vi "3D curvature tensor algebra --V3.vi"(5 "error mode":T1, 6 "means":T2, 7 "2D tensor action":T4, 9 "3D curvature Matrix IN":T3, 11 "3D curvature tensor IN":T5={"curvature Matrix"=[[3.0, 1.0], [1.0, 4.0]], "eigenvs"=[4.618033988749895, 2.381966011250105], "Eigenvectors"=[[-0.8506508083520399+0.0i, -0.5257311121191335+0.0i], [0.5257311121191335+0.0i, -0.8506508083520399+0.0i]], "theta (rad)"=0.5535743588970453, "theta (deg)"=31.717474411461012, "Δs"=[4.618033988749895, 2.381966011250105], "δG/G"=0.5535743588970453, "Δlog(s)"=[4.618033988749895, 2.381966011250105], "inverse Matrix"=[[3.0, 1.0], [1.0, 4.0]], "noise T"=0.5535743588970453} {"noise T" format="%#_3f"; "inverse Matrix" format="%#_3p"; "Δlog(s)" scale=0.001..10.0; "δG/G" format="%#_3f"; "Δs" format="%#_2p"; "theta (deg)" format="%#_3p"; "curvature Matrix" format="%#_3p"; "eigenvs" format="%#_2f"; "Eigenvectors" format="%#_3p"; "theta (rad)" format="%#_3p"}) -> (1 "3D curvature Matrix OUT":T3, 3 "3D curvature tensor OUT":T5={"curvature Matrix"=[[3.0, 1.0], [1.0, 4.0]], "eigenvs"=[4.618033988749895, 2.381966011250105], "Eigenvectors"=[[-0.8506508083520399+0.0i, -0.5257311121191335+0.0i], [0.5257311121191335+0.0i, -0.8506508083520399+0.0i]], "theta (rad)"=0.5535743588970453, "theta (deg)"=31.717474411461012, "Δs"=[4.618033988749895, 2.381966011250105], "δG/G"=0.5535743588970453, "Δlog(s)"=[4.618033988749895, 2.381966011250105], "inverse Matrix"=[[3.0, 1.0], [1.0, 4.0]], "noise T"=0.5535743588970453} {"noise T" format="%#_3f"; "inverse Matrix" format="%#_3p"; "Δlog(s)" scale=0.001..10.0; "δG/G" format="%#_3f"; "Δs" format="%#_2p"; "theta (deg)" format="%#_3p"; "curvature Matrix" format="%#_3p"; "eigenvs" format="%#_2f"; "Eigenvectors" format="%#_3p"; "theta (rad)" format="%#_3p"})   [LabVIEW 2021]
uses:
  3D curvature tensor.ctl
  <vilib>/Analysis/Matrix/Datatypes/RealMatrix.ctl
  <vilib>/Analysis/Matrix/Datatypes/ComplexMatrix.ctl
  2D curvature tensor actions.ctl
  3-vec.ctl
  nanocal generate curvature ellipse -- action.ctl
  <vilib>/Analysis/7linalg.llb/Eigenvalue and Vectors Output Option.ctl
  <vilib>/Analysis/7linalg.llb/Real Eigenvalues and Vectors.vi
  <vilib>/Analysis/baseanly.llb/Real Inverse Matrix.vi
  <vilib>/Analysis/NI_AALBase.lvlib
  <vilib>/Analysis/NI_AALPro.lvlib
  <vilib>/Analysis/Matrix/NI_Matrix.lvlib
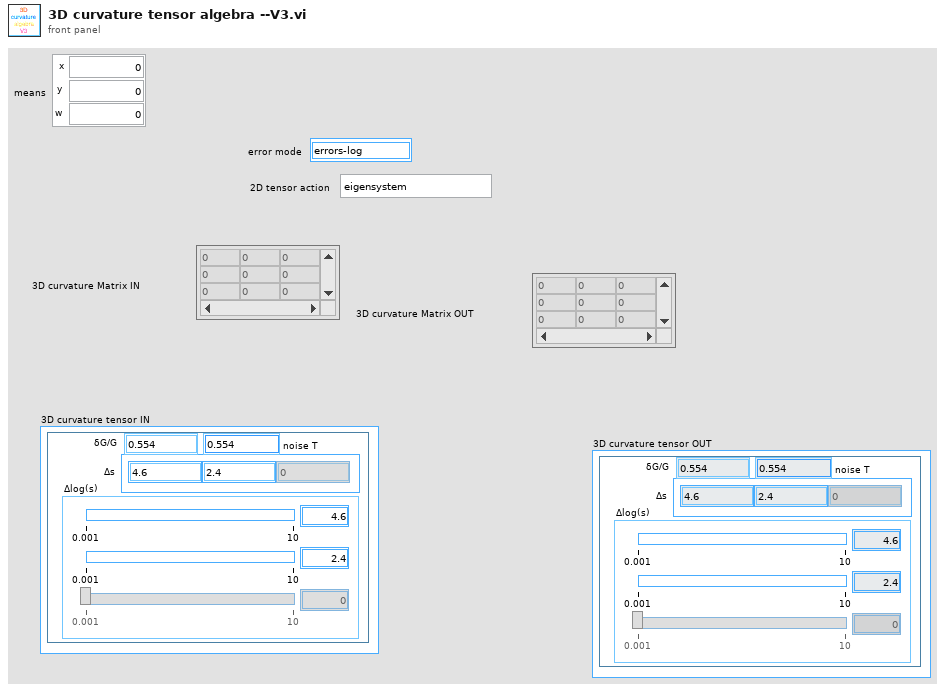
[diagram p1: front panel]
types:
  T1 = typedef "nanocal generate curvature ellipse -- action.ctl" = enum16{"errors-log", "errors-linear"}
  T2 = typedef "3-vec.ctl" = cluster{"x":dbl, "y":dbl, "w":dbl}
  T3 = typedef "NI_Matrix.lvlib/RealMatrix.ctl" = dbl[][]
  T4 = typedef "2D curvature tensor actions.ctl" = enum16{"eigensystem", "sigma", "set matrix", "inverse"}
  T5 = typedef "3D curvature tensor.ctl" = cluster{"curvature Matrix":T3, "eigenvs":dbl[], "Eigenvectors":T6, "theta (rad)":dbl, "theta (deg)":dbl, "Δs":dbl[], "δG/G":dbl, "Δlog(s)":dbl[], "inverse Matrix":T3, "noise T":dbl}
  T6 = typedef "NI_Matrix.lvlib/ComplexMatrix.ctl" = cdb[][]
  T7 = typedef "NI_AALPro.lvlib/Eigenvalue and Vectors Output Option.ctl" = i32
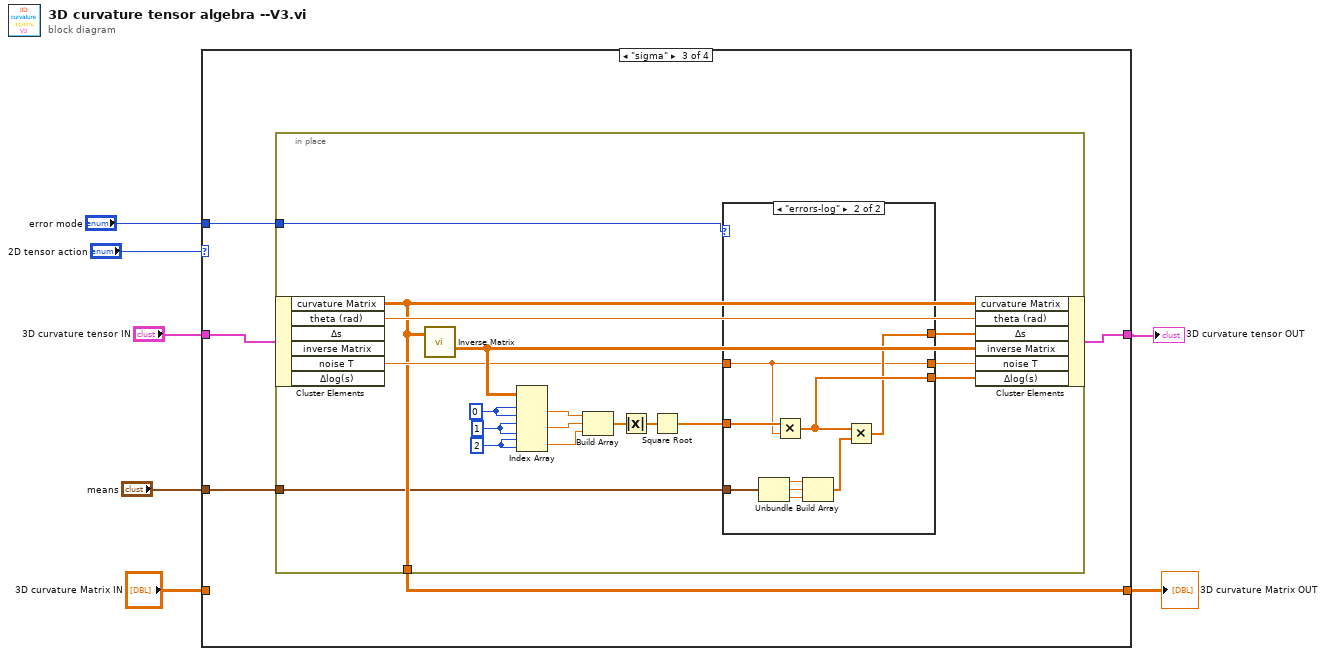
[diagram p0: block diagram]
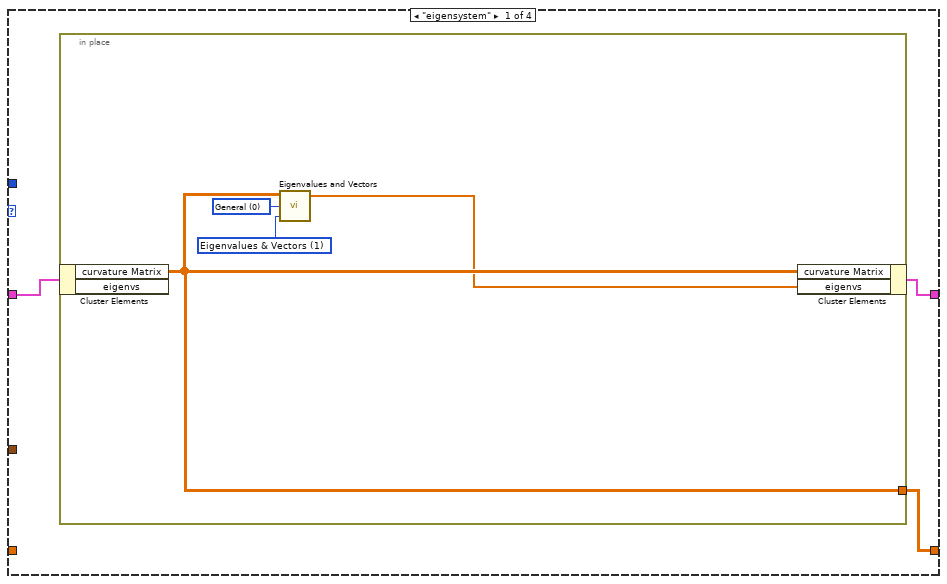
[diagram p2: hidden frame]
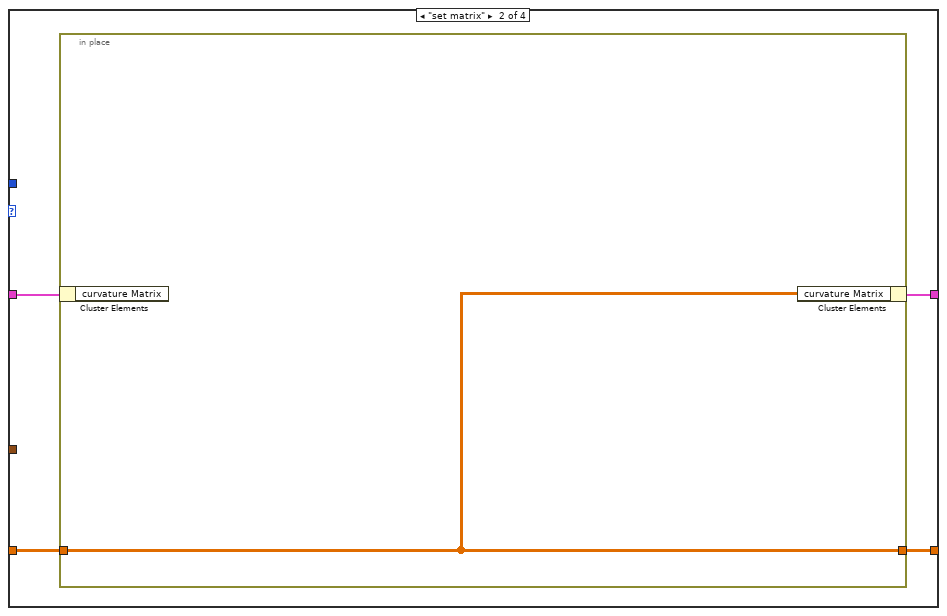
[diagram p3: hidden frame]
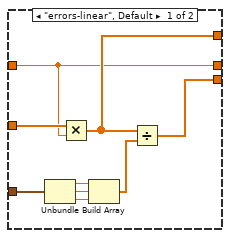
[diagram p4: hidden frame]
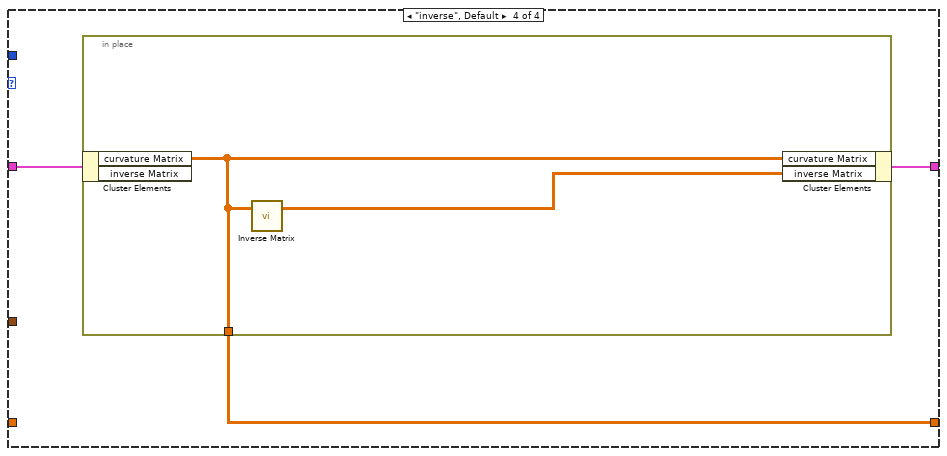
[diagram p5: hidden frame]
diagram:
  n1 = case shown="\"sigma\"" "2D tensor action" {
    tunnel: [w8 w17 w23 w62] -> w6
    tunnel: "3D curvature tensor IN" -> [w10 w18 w24 w63]
    tunnel: [w9 w16 w22 w61] -> w4
    tunnel: "3D curvature Matrix IN" -> [_ w15 _ _]
    tunnel: "means" -> [_ _ w21 _]
    tunnel: "error mode" -> [_ _ w20 _]
    frame "eigensystem" {
      n2 = in-place {
        in-place-border: [w14] -> w9
        w12 = T7 1 items=["Eigenvalues", "Eigenvalues & Vectors"] ("output option")
        w13 = 0 items=["General", "Symmetric"] ("matrix type")
        n3 = in-place-cluster #1(w10) -> ("curvature Matrix"=w14:T3)  [unwired: 1 out]
        n4 = call-poly <vilib>:"Eigenvalues and Vectors.vi"("output option"=w12, "matrix type"=w13, "Input Matrix"=w14) -> ("Eigenvalues"=w11:cdb[])  [unwired: 2 out]
        n5 = in-place-cluster #1("curvature Matrix"=w14, "eigenvs"=w11) -> (w8:T5)
      }
    }
    frame "set matrix" {
      n6 = in-place {
        in-place-border: [w19] -> w16
        in-place-border: w15 -> [w19]
        n7 = in-place-cluster #2(w18) -> ()  [unwired: 1 out]
        n8 = in-place-cluster #2("curvature Matrix"=w19) -> (w17:T5)
      }
    }
    frame "sigma" {
      n9 = in-place {
        in-place-border: [w30] -> w22
        in-place-border: w21 -> [w29]
        in-place-border: w20 -> [w26]
        w32 = 2 ("index (row)")
        w38 = 1 ("index")
        w39 = 0 ("index")
        n10 = in-place-cluster #3(w24) -> ("curvature Matrix"=w30:T3, "theta (rad)"=w42:dbl, "noise T"=w37:dbl)  [unwired: 3 out]
        n11 = call-poly <vilib>:"Inverse Matrix.vi"("Input Matrix"=w30) -> ("Inverse Matrix"=w40:T3)  [unwired: 1 in, 1 out]
        n12 = Index Array(array=w40, index (row) #1=w39, index (col) #1=w39, index (row) #2=w38, index (col) #2=w38, index (row) #3=w32, index (col) #3=w32) -> (element #1=w36:dbl, element #2=w35:dbl, element #3=w31:dbl)
        n13 = Build Array(w36, w35, w31) -> (w41:dbl[])
        n14 = Absolute Value(x=w41) -> (abs(x)=w33:dbl[])
        n15 = Square Root(x=w33) -> (sqrt(x)=w34:dbl[])
        n16 = case shown="\"errors-log\"" w26 {
          tunnel: w37 -> [w43 w52]
          tunnel: w34 -> [w51 w60]
          tunnel: w29 -> [w50 w59]
          tunnel: [w46 w53] -> w28
          tunnel: [w44 w54] -> w27
          tunnel: [w43 w52] -> w25
          frame "errors-linear", Default {
            n17 = Unbundle(w50) -> ("x"=w49:dbl, "y"=w48:dbl, "w"=w47:dbl)
            n18 = Multiply(x=w51, y=w43) -> (x*y=w46:dbl[])
            n19 = Build Array(w49, w48, w47) -> (w45:dbl[])
            n20 = Divide(x=w46, y=w45) -> (x/y=w44:dbl[])
          }
          frame "errors-log" {
            n21 = Unbundle(w59) -> ("x"=w58:dbl, "y"=w57:dbl, "w"=w56:dbl)
            n22 = Multiply(x=w60, y=w52) -> (x*y=w54:dbl[])
            n23 = Build Array(w58, w57, w56) -> (w55:dbl[])
            n24 = Multiply(x=w54, y=w55) -> (x*y=w53:dbl[])
          }
        }
        n25 = in-place-cluster #3("curvature Matrix"=w30, "theta (rad)"=w42, "Δs"=w28, "inverse Matrix"=w40, "noise T"=w25, "Δlog(s)"=w27) -> (w23:T5)
      }
    }
    frame "inverse", Default {
      n26 = in-place {
        in-place-border: [w64] -> w61
        n27 = in-place-cluster #4(w63) -> ("curvature Matrix"=w64:T3)  [unwired: 1 out]
        n28 = call-poly <vilib>:"Inverse Matrix.vi"("Input Matrix"=w64) -> ("Inverse Matrix"=w65:T3)  [unwired: 1 in, 1 out]
        n29 = in-place-cluster #4("curvature Matrix"=w64, "inverse Matrix"=w65) -> (w62:T5)
      }
    }
  }
  "3D curvature tensor OUT" <- w6
  "3D curvature Matrix OUT" <- w4
